vi "sub 2.vi"(8 "error in (no error)":errorcluster, 10 "Data to Log":dbl[][](array[numeric]), 11 "File Refnum In":refnum<file>) -> (0 "error out":errorcluster, 3 "File Refnum Out":refnum<file>)   [LabVIEW 2015]
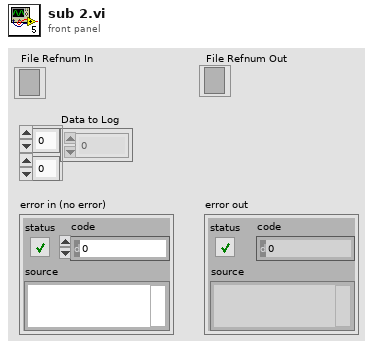
[diagram p1: front panel]
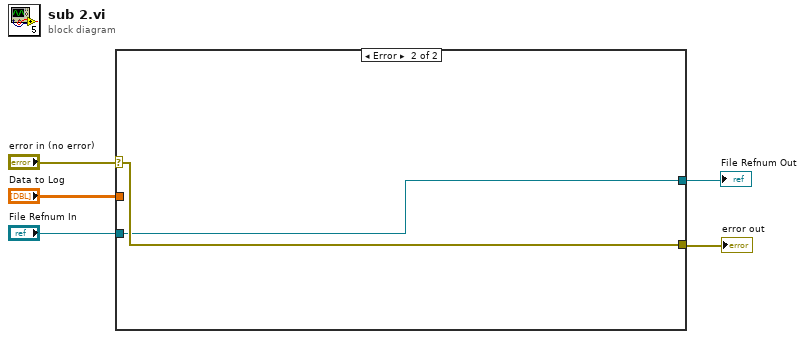
[diagram p0: block diagram]
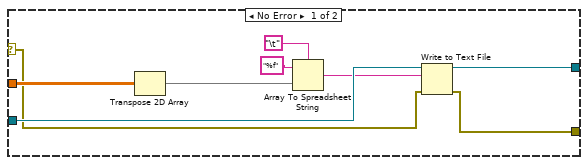
[diagram p2: hidden frame]
diagram:
  n1 = case shown="Error" "error in (no error)" {
    selector: "error in (no error)" -> [w7 w16]
    tunnel: "Data to Log" -> [w14 _]
    tunnel: "File Refnum In" -> [w12 w15]
    tunnel: [w11 w15] -> w3
    tunnel: [w6 w16] -> w5
    frame No Error {
      n2 = Transpose 2D Array(2D array=w14) -> (transposed array=w13:dbl[][])
      n3 = Array To Spreadsheet String(delimiter (Tab)="\t", array=w13, 3:"%f" ("format string")) -> (spreadsheet string=w8:string)
      n4 = Write to Text File(file (use dialog)=w12, text=w8, error in=w7) -> (refnum out=w11:refnum<file>, error out=w6:errorcluster)  [unwired: 1 in, 1 out]
    }
    frame Error {
    }
  }
  "File Refnum Out" <- w3
  "error out" <- w5
